vi "Increment or decrement.vi"(10 "Increment/Decrement value":u64, 11 "SubscriptionDetailsParent in":refnum<class "SubscriptionDetailsParent.lvclass">) -> (3 "SubscriptionDetailsParent out":refnum<class "SubscriptionDetailsParent.lvclass">)   [LabVIEW 2020, in "wamplv.lvlib" / "SubscriptionDetailsParent.lvclass"]
uses:
  SubscriptionDetailsParent.lvclass
  SubscriptionDetailsParent.lvclass/SubscriptionDetailsParent.ctl
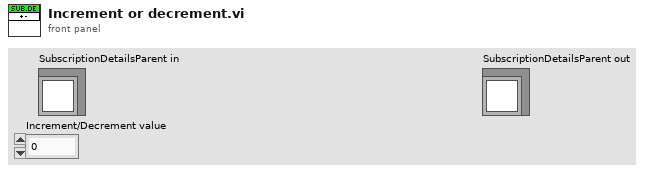
[diagram p1: front panel]
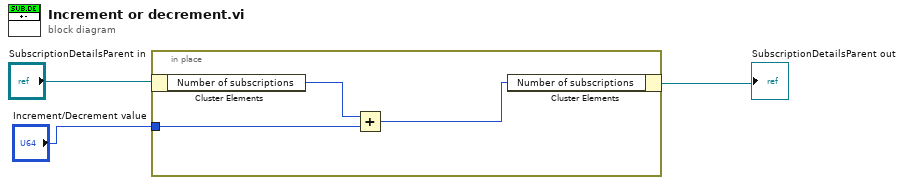
[diagram p0: block diagram]
diagram:
  n1 = in-place {
    in-place-border: "Increment/Decrement value" -> [w5]
    n2 = in-place-cluster #1("SubscriptionDetailsParent in") -> ("Number of subscriptions"=w6:u64)
    n3 = Add(x=w6, y=w5) -> (x+y=w4:u64)
    n4 = in-place-cluster #1("Number of subscriptions"=w4) -> (→"SubscriptionDetailsParent out":refnum<class "SubscriptionDetailsParent.lvclass">)
  }
